vi "Match Axis NEW (SubVI).vi"(0 "Axis ID":string, 7 "input string":string, 9 "Visa name in":refnum<visa-resource-name>, 11 "error in":errorcluster) -> (2 "Good\nto read!":bool, 4 "out number":dbl, 8 "out string":string, 10 "Visa name out":refnum<visa-resource-name>, 13 "status":bool, 15 "error out":errorcluster)   [LabVIEW 2013]
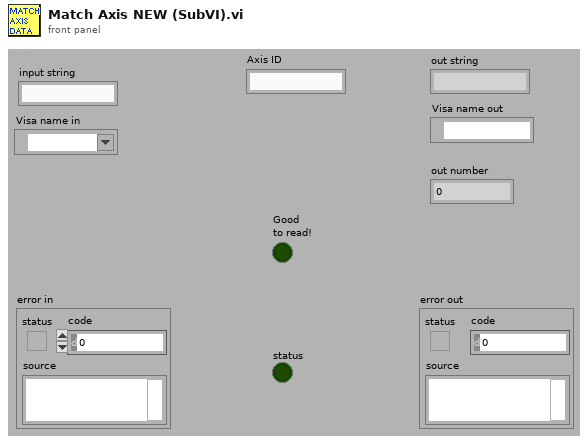
[diagram p1: front panel]
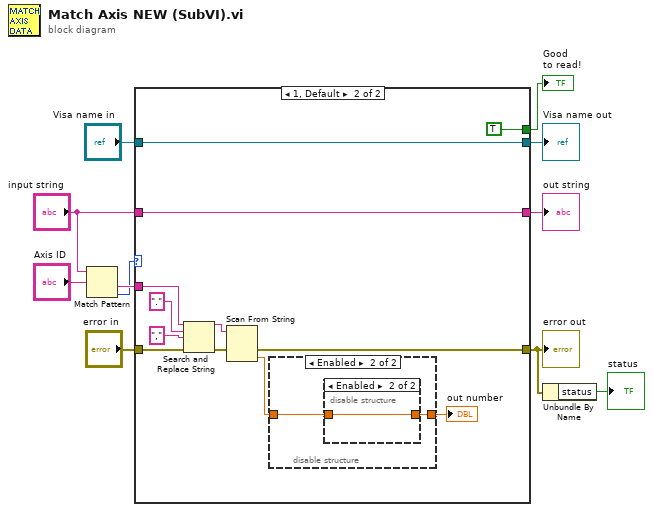
[diagram p0: block diagram]
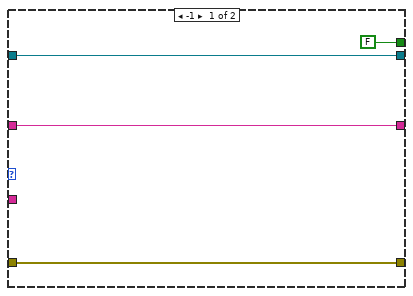
[diagram p2: hidden frame]
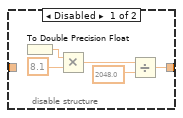
[diagram p3: hidden frame]
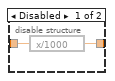
[diagram p4: hidden frame]
diagram:
  n1 = Match Pattern(string="input string", regular expression="Axis ID") -> (after substring=w8:string, offset past match=w7:i32)  [unwired: 3 out]
  n2 = case shown="1, Default" w7 {
    tunnel: [w15 w23] -> w5
    tunnel: w8 -> [_ w21]
    tunnel: "error in" -> [w15 w17]
    tunnel: "Visa name in" -> [w14 w27]
    tunnel: [w14 w27] -> w11
    tunnel: [w13 w26] -> w2
    tunnel: "input string" -> [w13 w26]
    tunnel: [FALSE ("status") TRUE ("status")] -> w1
    frame -1 {
    }
    frame 1, Default {
      n3 = Search and Replace String(input string=w21, search string=".", replace string="," ("search string"), error in=w17) -> (result string=w20:string, error out=w16:errorcluster)  [unwired: 6 out]
      n4 = Scan From String(input string=w20, error in=w16) -> (error out=w23:errorcluster, output 1=w22:dbl)  [unwired: 3 in, 2 out]
      n5 = disable-structure shown="Enabled" {
        disable-tunnel: [w29 w33] -> w25
        disable-tunnel: w22 -> [_ w34]
        frame Disabled {
          n6 = To Double Precision Float() -> (double precision float=w30:dbl)  [unwired: 1 in]
          n7 = Multiply(x=w30, y=8.1) -> (x*y=w32:dbl)
          n8 = Divide(x=w32, y=2048.0) -> (x/y=w29:dbl)
        }
        frame Enabled {
          n9 = disable-structure shown="Enabled" {
            disable-tunnel: w34 -> [w36 w37]
            disable-tunnel: [w35 w37] -> w33
            frame Disabled {
              n10 = expression code="x/1000"(w36) -> (w35:dbl)
            }
            frame Enabled {
            }
          }
        }
      }
      "out number" <- w25
    }
  }
  "Visa name out" <- w11
  "error out" <- w5
  "out string" <- w2
  "Good\nto read!" <- w1
  n11 = Unbundle By Name(w5) -> ("status"=→"status":bool)
